vi "Property Tree Symbol Handler_2.vi"(7 "Save Action":T1=enum."Wire Unbundle", 11 "Tree refs":refnum<vi>[](array[refnum])) -> ()   [LabVIEW 2023]
doc: "Synchronize scroll position and value of registered tree controls."
uses:
  controls/action enum.ctl
panel:
  out "Clicked Item Disabled":bool
  out "Double Click":bool
  out "Source":u32(ring) items=["LabVIEW UI"=0, "ActiveX"=1, "User Event"=25]
  in  "Main Tree":string[](tree)
  in  "Write Tree":string[](tree)
  in  "Read Tree":string[](tree)
  in  "Stop":bool
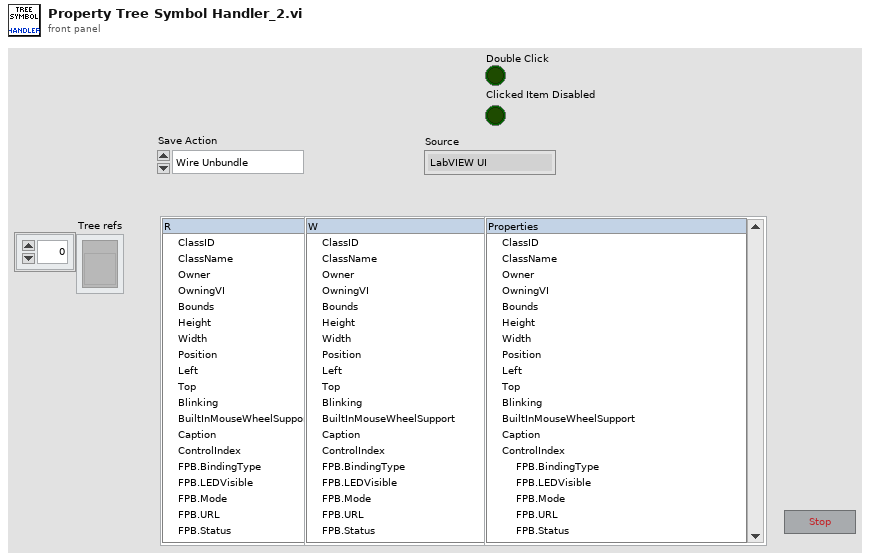
[diagram p1: front panel]
types:
  T1 = typedef "action enum.ctl" = enum16{"[NONE]", "APP_SEPARATOR", "Wire Bundle", "Wire Unbundle", "Terminal Unbundle", "Terminal Bundle", "Bundler Move Up", "Bundler Move Down", "Bundler Insert", "Bundler Remove", "Bundler Remove Unwired", "Bundler Rearrange", "In Place Insert", "In Place Remove", "In Place Remove Unwired", "In Place Rearrange", "Wire Properties", "Wire Method", "Terminal Properties", "Terminal Method", "Property Move Up", "Property Move Down", "Properties Insert", "Properties Remove", "Properties Remove Unwired", "Properties Rearrange", "Method Change", "Class For Constant", "Class For Control", "Class For Node", "Class Name to Clipboard"}
  T2 = enum16{"Init", "Read", "Remove", "Remove or Append", "Append", "Append If New"}
  T3 = cluster{"Tag":string, "Read":bool, "Write":bool, "New":bool}
  T4 = cluster{"Tag":string, "Read":bool, "Write":bool, "New":bool}[]
  T5 = typedef "LVPoint32TypeDef.ctl" = cluster{"Horizontal":i32, "Vertical":i32}
  T6 = typedef "eventsource.ctl" = u32
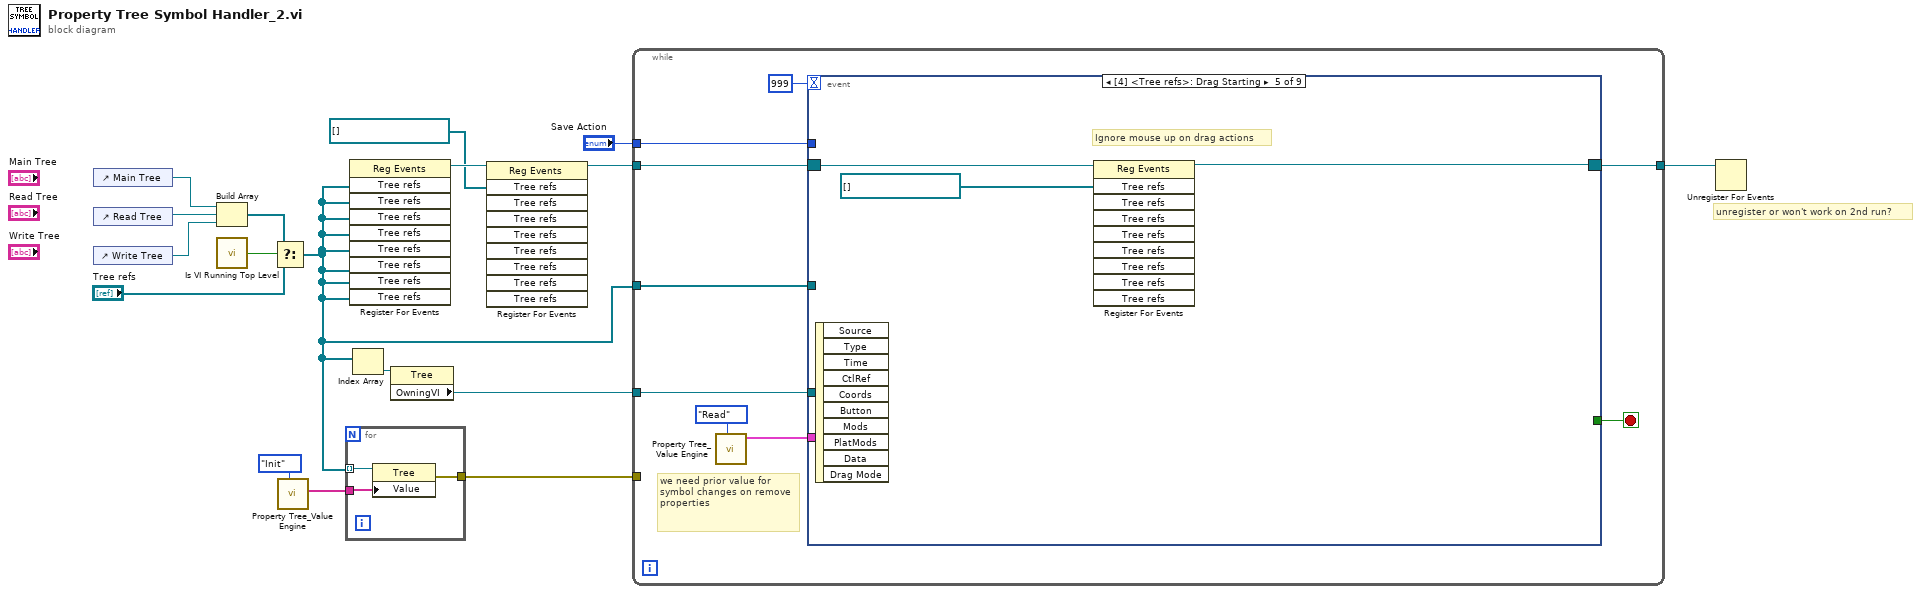
[diagram p0: block diagram]
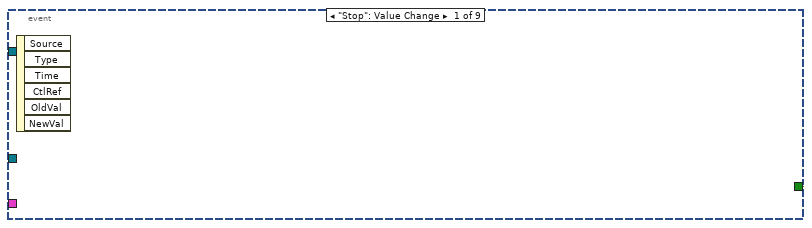
[diagram p2: hidden frame]
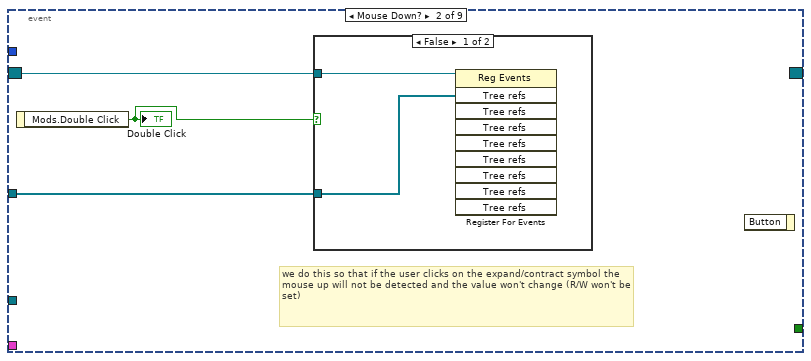
[diagram p3: hidden frame]
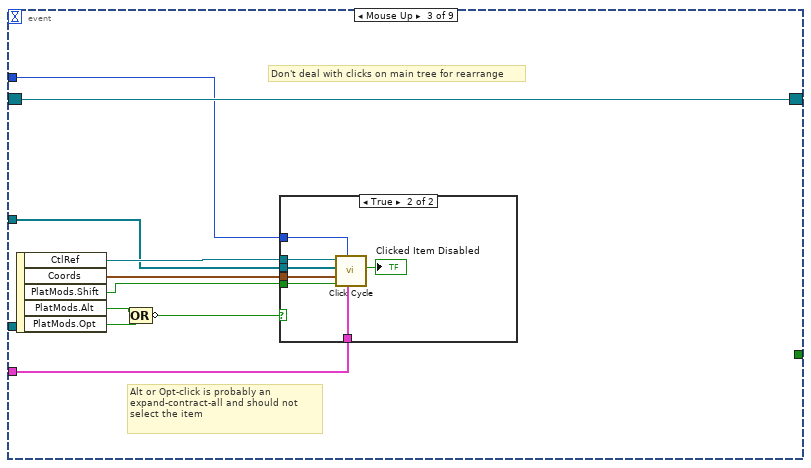
[diagram p5: hidden frame]
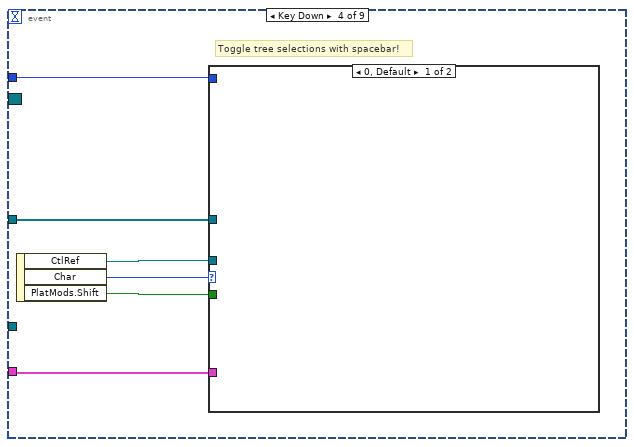
[diagram p7: hidden frame]
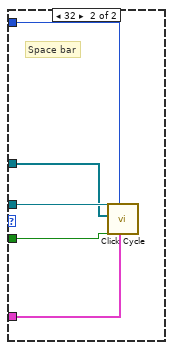
[diagram p8: hidden frame]
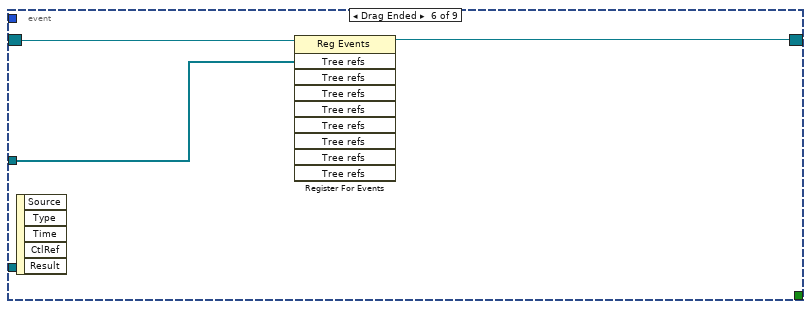
[diagram p9: hidden frame]
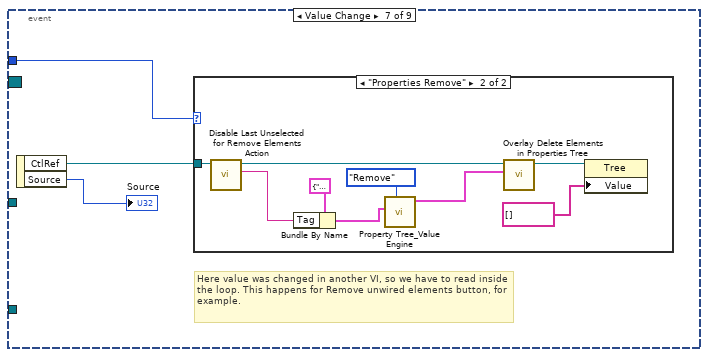
[diagram p10: hidden frame]
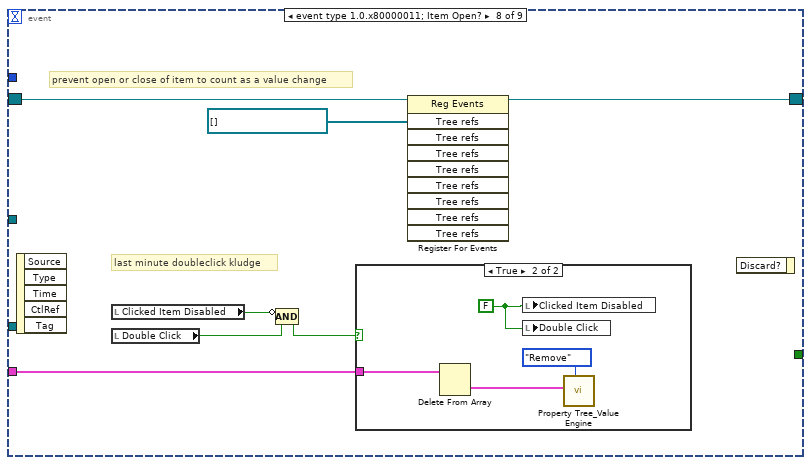
[diagram p12: hidden frame]
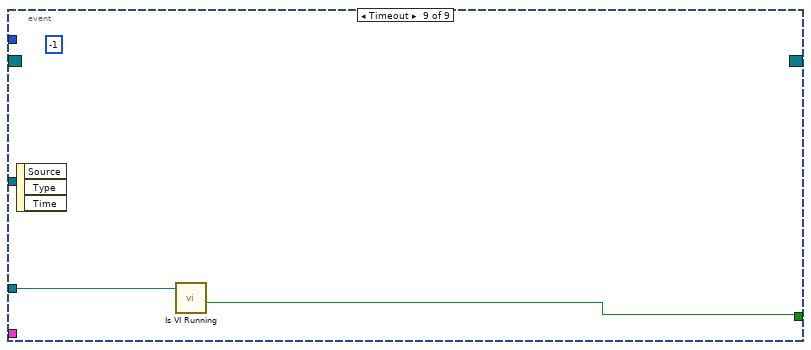
[diagram p14: hidden frame]
diagram:
  # "unregister or won't work on 2nd run?"
  n1 = control-ref of="Main Tree"() -> (w2:refnum<vi>)
  n2 = control-ref of="Read Tree"() -> (w17:refnum<vi>)
  n3 = control-ref of="Write Tree"() -> (w16:refnum<vi>)
  n4 = Build Array(w2, w17, w16) -> (w15:refnum<vi>[])
  n5 = call "Is VI Running Top Level.vi"() -> ("Top Level?"=w7:bool)  [unwired: 5 in]
  n6 = Select(t=w15, s=w7, f="Tree refs") -> (s? t:f=w1:refnum<vi>[])
  n7 = call "Property Tree_Value Engine.vi"("Save Action"=T2."Init" ("Action")) -> ("Tag Array"=w10:string[])  [unwired: 8 in, 2 out]
  n8 = for {
    tunnel: w10 -> [w19]
    tunnel: w1 -> [w20] mode=indexing
    tunnel: [w18] -> w9
    n9 = property class="Tree"(reference=w20, "Value"=w19) -> (error out=w18:errorcluster)  [unwired: 1 in, 1 out]
  }
  n10 = register-events(w1, w1, w1, w1, w1, w1, w1, w1) -> (reference out=w5:refnum<event-registration>)  [unwired: 2 in, 1 out]
  n11 = Index Array(array=w1) -> (element=w13:refnum<vi>)  [unwired: 1 in]
  n12 = property class="Tree"(reference=w13) -> ("OwningVI"=w12:refnum<vi>)  [unwired: 1 in, 2 out]
  n13 = register-events(reference=w5, refnum<vi>[] [] ("event source")) -> (reference out=w4:refnum<event-registration>)  [unwired: 8 in, 1 out]
  n14 = while {
    tunnel: w4 -> [w28]
    tunnel: w12 -> [w27]
    tunnel: w1 -> [w26]
    tunnel: w9 -> [_]
    tunnel: "Save Action" -> [w25]
    tunnel: [w24] -> w6
    stop <- w29 stop-if-true
    # "we need prior value for symbol changes on remove properties"
    n15 = call "Property Tree_Value Engine.vi"("Save Action"=T2."Read" ("Action")) -> ("Property Array Out"=w22:T4)  [unwired: 8 in, 2 out]
    n16 = event shown="[4] <Tree refs>: Drag Starting" {
      selector: w28 -> [_ w33 w45 _ w66 w69 _ w88 _]
      dyn-events: [_ _ w45 _ w65 w68 _ w87 _] -> w24
      timeout: 999 -> [_ _ _ _ _ _ _ _ _]
      tunnel: ["Stop" _ _ _ _ _ _ _ w93] -> w29
      tunnel: w27 -> [_ _ _ _ _ _ _ _ w94]
      tunnel: w26 -> [_ w32 w42 w56 _ w67 _ _ _]
      tunnel: w25 -> [_ _ w40 w55 _ _ w71 _ _]
      tunnel: w22 -> [_ _ w41 w53 _ _ _ w85 _]
      event "Stop": Value Change {
        n17 = event-data() -> ()  [unwired: 1 in, 6 out]
      }
      event Mouse Down? {
        # "we do this so that if the user clicks on the expand/contract symbol the mouse up will not be detected and the value won't change (R/W won't be set)"
        n18 = event-data() -> ("Mods.Double Click"=w31:bool)  [unwired: 1 in]
        "Double Click" <- w31
        n19 = case shown="False" w31 {
          tunnel: w33 -> [w35 _]
          tunnel: w32 -> [w34 _]
          frame False {
            n20 = register-events(reference=w35, w34) -> ()  [unwired: 8 in, 2 out]
          }
          frame True {
          }
        }
        n21 = event-data() -> ()  [unwired: 2 in, 1 out]
      }
      event Mouse Up {
        # "Alt or Opt-click is probably an expand-contract-all and should not select the item"
        # "Don't deal with clicks on main tree for rearrange"
        n22 = event-data() -> ("CtlRef"=w44:refnum<vi>, "Coords"=w39:T5, "PlatMods.Shift"=w43:bool, "PlatMods.Alt"=w38:bool, "PlatMods.Opt"=w37:bool)  [unwired: 1 in]
        n23 = Compound Arithmetic op=OR(w38, w37) -> (invert w36:bool)
        n24 = case shown="True" w36 {
          tunnel: w44 -> [_ w52]
          tunnel: w43 -> [_ w51]
          tunnel: w42 -> [_ w50]
          tunnel: w41 -> [_ w49]
          tunnel: w40 -> [_ w48]
          tunnel: w39 -> [_ w47]
          frame False {
          }
          frame True {
            n25 = call "Click Cycle.vi"("Prior Property Selection"=w49, "Action"=w48, "Shift"=w51, "Coords"=w47, "All Tree Refs"=w50, "Tree Control Ref"=w52) -> ("Clicked disabled item?"=→"Clicked Item Disabled":bool)  [unwired: 4 in, 1 out]
          }
        }
      }
      event Key Down {
        # "Toggle tree selections with spacebar!"
        n26 = event-data() -> ("CtlRef"=w57:refnum<vi>, "Char"=w58:i16, "PlatMods.Shift"=w54:bool)  [unwired: 1 in]
        n27 = case shown="0, Default" w58 {
          tunnel: w57 -> [_ w63]
          tunnel: w56 -> [_ w62]
          tunnel: w55 -> [_ w61]
          tunnel: w54 -> [_ w60]
          tunnel: w53 -> [_ w59]
          frame 0, Default {
          }
          frame 32 {
            # "Space bar"
            n28 = call "Click Cycle.vi"("Prior Property Selection"=w59, "Action"=w61, "Shift"=w60, "All Tree Refs"=w62, "Tree Control Ref"=w63) -> ()  [unwired: 5 in, 2 out]
          }
        }
      }
      event Drag Starting {
        # "Ignore mouse up on drag actions"
        n29 = event-data() -> ()  [unwired: 1 in, 10 out]
        n30 = register-events(reference=w66, refnum<vi>[] [] ("event source")) -> (reference out=w65:refnum<event-registration>)  [unwired: 8 in, 1 out]
      }
      event Drag Ended {
        n31 = event-data() -> ()  [unwired: 1 in, 5 out]
        n32 = register-events(reference=w69, w67) -> (reference out=w68:refnum<event-registration>)  [unwired: 8 in, 1 out]
      }
      event Value Change {
        # "Here value was changed in another VI, so we have to read inside the loop. This happens for Remove unwired elements button, for example."
        n33 = event-data() -> ("CtlRef"=w70:refnum<vi>, "Source"=→"Source":T6)  [unwired: 1 in]
        n34 = case shown="\"Properties Remove\"" w71 {
          tunnel: w70 -> [_ w80]
          frame Default {
          }
          frame "Properties Remove" {
            n35 = call "Disable Last Unselected for Remove Elements Action.vi"("Tree Ref"=w80) -> ("Removed Item Tag"=w73:string, "Tree Ref Out"=w81:refnum<vi>)  [unwired: 8 in, 1 out]
            n36 = Bundle By Name(cluster=T3 {"Tag"="", "Read"=FALSE, "Write"=FALSE, "New"=FALSE} ("Element"), "Tag"=w73) -> (w75:T3)
            n37 = call "Property Tree_Value Engine.vi"("Save Action"=T2."Remove" ("Action"), "Element"=w75) -> ("Property Array Out"=w76:T4)  [unwired: 7 in, 2 out]
            n38 = call "Overlay Delete Elements in Properties Tree.vi"("Prior Property Array"=w76, "Tree Ref"=w81) -> ("Tree Ref Out"=w79:refnum<vi>)  [unwired: 8 in, 1 out]
            n39 = property class="Tree"(reference=w79, "Value"=string[] []) -> ()  [unwired: 1 in, 2 out]
          }
        }
      }
      event event type 1.0.x80000011; Item Open? {
        # "last minute doubleclick kludge"
        # "prevent open or close of item to count as a value change"
        n40 = event-data() -> ()  [unwired: 1 in, 5 out]
        n41 = local read "Clicked Item Disabled"() -> (w84:bool)
        n42 = local read "Double Click"() -> (w83:bool)
        n43 = Compound Arithmetic op=AND(invert w84, w83) -> (w82:bool)
        n44 = case shown="True" w82 {
          tunnel: w85 -> [_ w90]
          frame False {
          }
          frame True {
            w89 = FALSE
            n45 = Delete From Array(array=w90) -> (deleted portion=w91:T3)  [unwired: 2 in, 1 out]
            n46 = local write "Clicked Item Disabled"(w89) -> ()
            n47 = local write "Double Click"(w89) -> ()
            n48 = call "Property Tree_Value Engine.vi"("Save Action"=T2."Remove" ("Action"), "Element"=w91) -> ()  [unwired: 7 in, 3 out]
          }
        }
        n49 = register-events(reference=w88, refnum<vi>[] [] ("event source")) -> (reference out=w87:refnum<event-registration>)  [unwired: 8 in, 1 out]
        n50 = event-data() -> ()  [unwired: 2 in, 1 out]
      }
      event Timeout {
        (unwired) -1
        n51 = event-data() -> ()  [unwired: 1 in, 3 out]
        n52 = call "Is VI Running.vi"("VI in"=w94) -> ("VI Not Running"=w93:bool)  [unwired: 7 in, 3 out]
      }
    }
  }
  n53 = Unregister For Events(event registration refnum=w6) -> ()  [unwired: 1 in, 1 out]
